vi "String - Convert Str (YYYYmmdd_HHMMSS) to TimeStamp.vi"(11 "YYYYmmdd_HHMMSS":string) -> (1 "DateTime Cluster":T1, 2 "time stamp":timestamp, 3 "YYYY-mm-dd HH:MM:SS":string)   [LabVIEW 2013]
uses:
  <vilib>/Utility/miscctls.llb/LVDateTimeRec.ctl
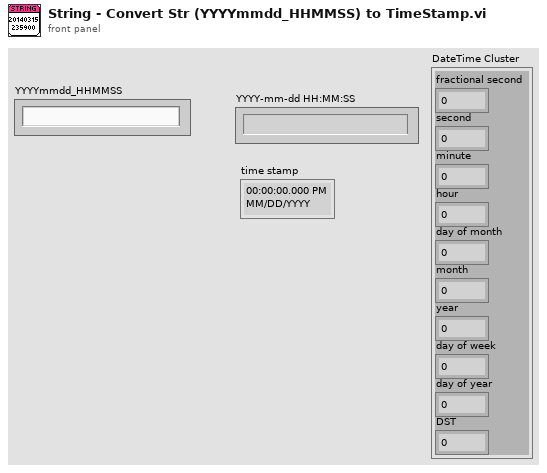
[diagram p1: front panel]
types:
  T1 = typedef "LVDateTimeRec.ctl" = cluster{"fractional second":dbl, "second":i32, "minute":i32, "hour":i32, "day of month":i32, "month":i32, "year":i32, "day of week":i32, "day of year":i32, "DST":i32}
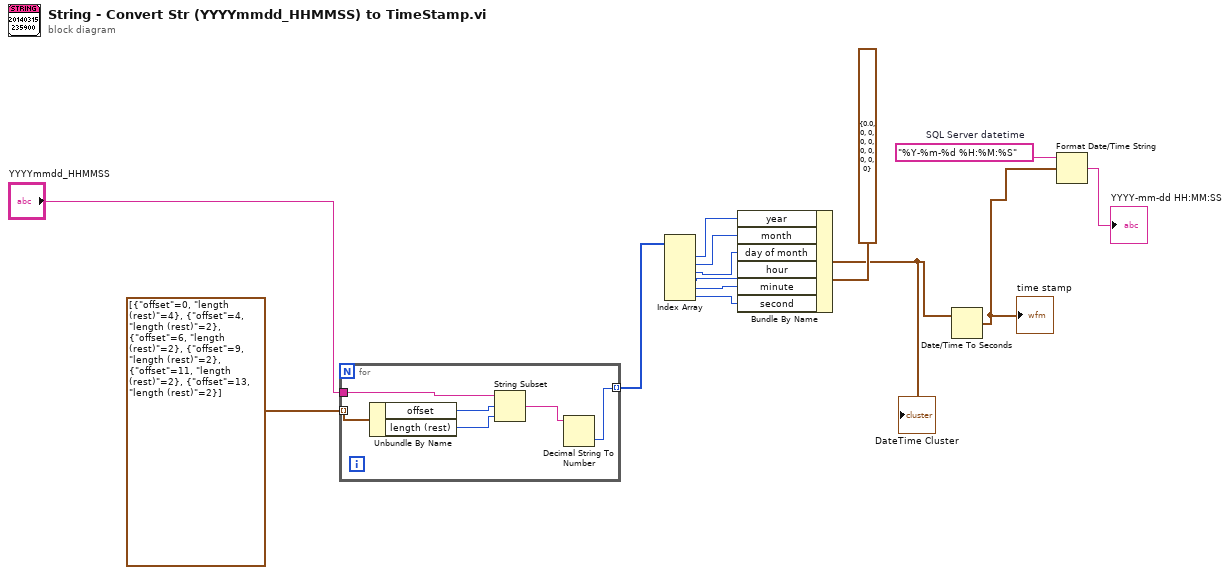
[diagram p0: block diagram]
diagram:
  w10 = "%Y-%m-%d %H:%M:%S"  # SQL Server datetime
  n1 = for {
    tunnel: "YYYYmmdd_HHMMSS" -> [w20]
    tunnel: cluster{"offset":i32, "length (rest)":i32}[] [{"offset"=0, "length (rest)"=4}, {"offset"=4, "length (rest)"=2}, {"offset"=6, "length (rest)"=2}, {"offset"=9, "length (rest)"=2}, {"offset"=11, "length (rest)"=2}, {"offset"=13, "length (rest)"=2}] -> [w19] mode=indexing
    tunnel: [w15] -> w9 mode=indexing
    n2 = Unbundle By Name(w19) -> ("offset"=w18:i32, "length (rest)"=w17:i32)
    n3 = String Subset(string=w20, offset (0)=w18, length (rest)=w17) -> (substring=w16:string)
    n4 = Decimal String To Number(string=w16) -> (number=w15:i32)  [unwired: 2 in, 1 out]
  }
  n5 = Index Array(array=w9) -> (element #1=w1:i32, element #2=w8:i32, element #3=w7:i32, element #4=w6:i32, element #5=w5:i32, element #6=w4:i32)  [unwired: 6 in]
  n6 = Bundle By Name(cluster=T1 {"fractional second"=0.0, "second"=0, "minute"=0, "hour"=0, "day of month"=0, "month"=0, "year"=0, "day of week"=0, "day of year"=0, "DST"=0} ("date time rec"), "year"=w1, "month"=w8, "day of month"=w7, "hour"=w6, "minute"=w5, "second"=w4) -> (w11:T1)
  "DateTime Cluster" <- w11
  n7 = Date/Time To Seconds(2:w11) -> (0:w3:timestamp)  [unwired: 1 in]
  "time stamp" <- w3
  n8 = Format Date/Time String(time format string (%c)=w10, seconds (now)=w3) -> (date/time string=→"YYYY-mm-dd HH:MM:SS":string)  [unwired: 1 in]
